vi "failIf.vi"(7 "custom report message (\"\")":string, 8 "error in (no error)":errorcluster, 9 "message (\"\")":string, 10 "fail":bool, 11 "TestCase in":refnum<class "TestCase.lvclass">) -> (0 "error out":errorcluster, 3 "TestCase out":refnum<class "TestCase.lvclass">)   [LabVIEW 2011, in "TestCase.lvclass"]
doc: "Fail if 'fail' condition is TRUE. On failure, 'message' is appended to failure status."
uses:
  TestCase.lvclass
  TestCase.lvclass/TestCase.ctl
panel:
  # "JKI VI Tester for LabVIEW\nhttp://jkisoft.com/vi-tester\nCopyright (C) 2007-2009, JKI <info@jkisoft.com>\nALL RIGHTS RESERVED"
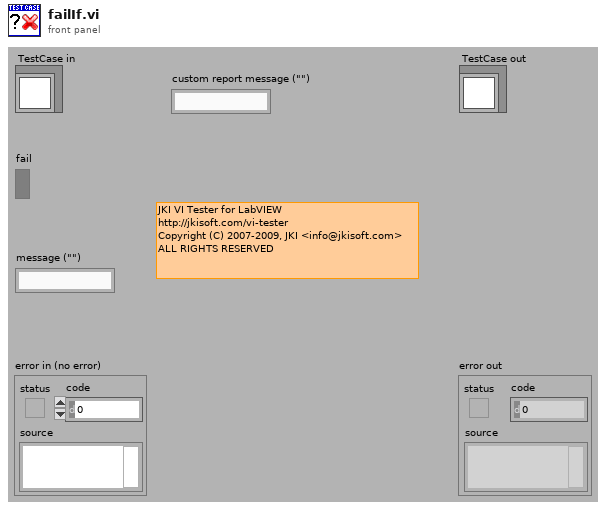
[diagram p1: front panel]
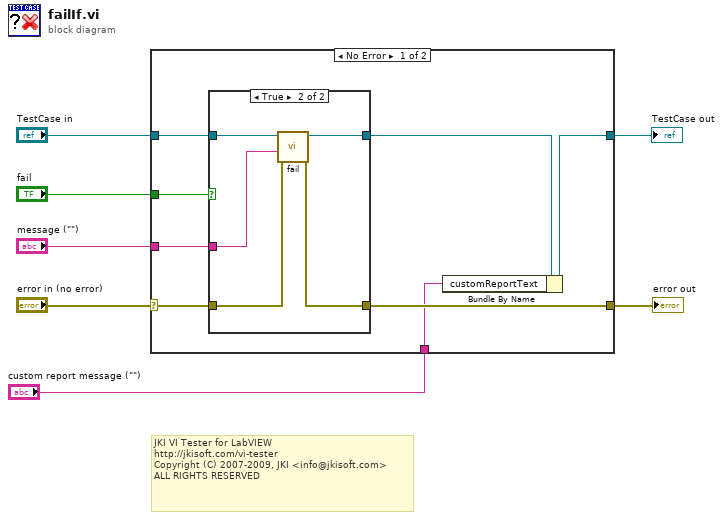
[diagram p0: block diagram]
diagram:
  # "JKI VI Tester for LabVIEW\nhttp://jkisoft.com/vi-tester\nCopyright (C) 2007-2009, JKI <info@jkisoft.com>\nALL RIGHTS RESERVED"
  n1 = case shown="No Error" "error in (no error)" {
    selector: "error in (no error)" -> [w15 w24]
    tunnel: [w14 w24] -> w6
    tunnel: [w9 w23] -> w4
    tunnel: "TestCase in" -> [w11 w23]
    tunnel: "message (\"\")" -> [w13 _]
    tunnel: "fail" -> [w12 _]
    tunnel: "custom report message (\"\")" -> [w8 _]
    frame No Error {
      n2 = case shown="True" w12 {
        tunnel: w15 -> [w17 w22]
        tunnel: [w17 w21] -> w14
        tunnel: w13 -> [_ w20]
        tunnel: w11 -> [w16 w19]
        tunnel: [w16 w18] -> w10
        frame False {
        }
        frame True {
          n3 = call-dynamic "fail.vi"("error in (no error)"=w22, "message (\"\")"=w20, "TestCase in"=w19) -> ("error out"=w21:errorcluster, "TestCase out"=w18:refnum<class "TestCase.lvclass">)  [unwired: 7 in]
        }
      }
      n4 = Bundle By Name(cluster=w10, "customReportText"=w8) -> (w9:refnum<class "TestCase.lvclass">)
    }
    frame Error {
    }
  }
  "error out" <- w6
  "TestCase out" <- w4
